vi "ETRONzipSummary.vi"() -> ()   [LabVIEW 2012]
uses:
  <vilib>/addons/database/Connection.llb/DB Tools Open Connec (Path).vi
  <vilib>/addons/database/Connection.llb/Conn Execute.vi
  <vilib>/addons/database/Recordset.llb/Rec Fetch Integer Data (R).vi
  <vilib>/addons/database/Recordset.llb/Rec Destroy - Connection.vi
  <vilib>/Utility/SMTP/NI_SMTPEmail.lvlib
  <vilib>/addons/database/NI_Database_API.lvlib
panel:
  out "concatenated string":string
  out "error out":errorcluster
  out "error out 3":errorcluster
  in  "MIME content-type (application/octet-stream)":string="application/octet-stream"
  out "error out 2":errorcluster
  out "last mod":timestamp
  in  "path":path=path "C:/temp/ETRON"
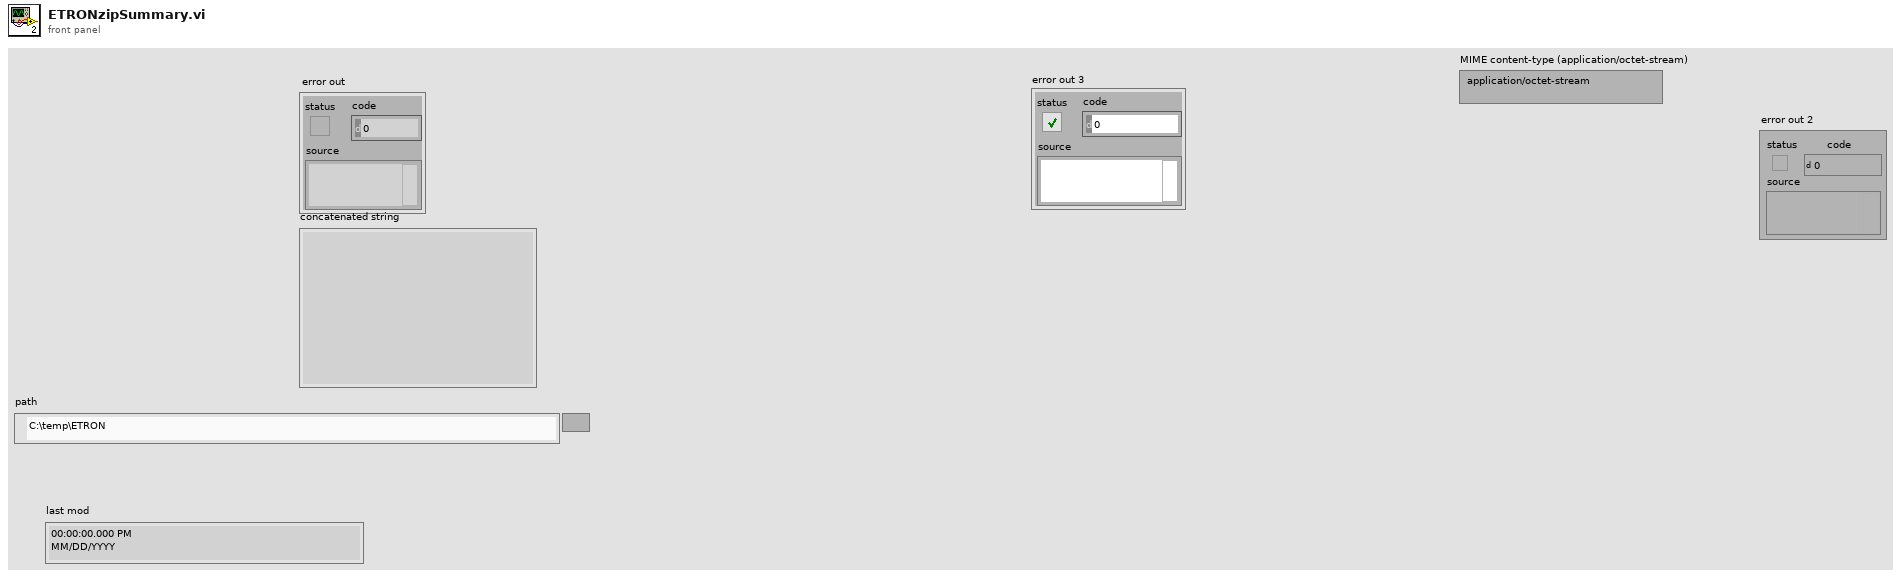
[diagram p1: front panel]
types:
  T1 = typedef "NI_Database_API.lvlib/Conn ObjectReference.ctl" = refnum<k1>
  T2 = typedef "NI_Database_API.lvlib/Rec ObjectReference.ctl" = refnum<k1>
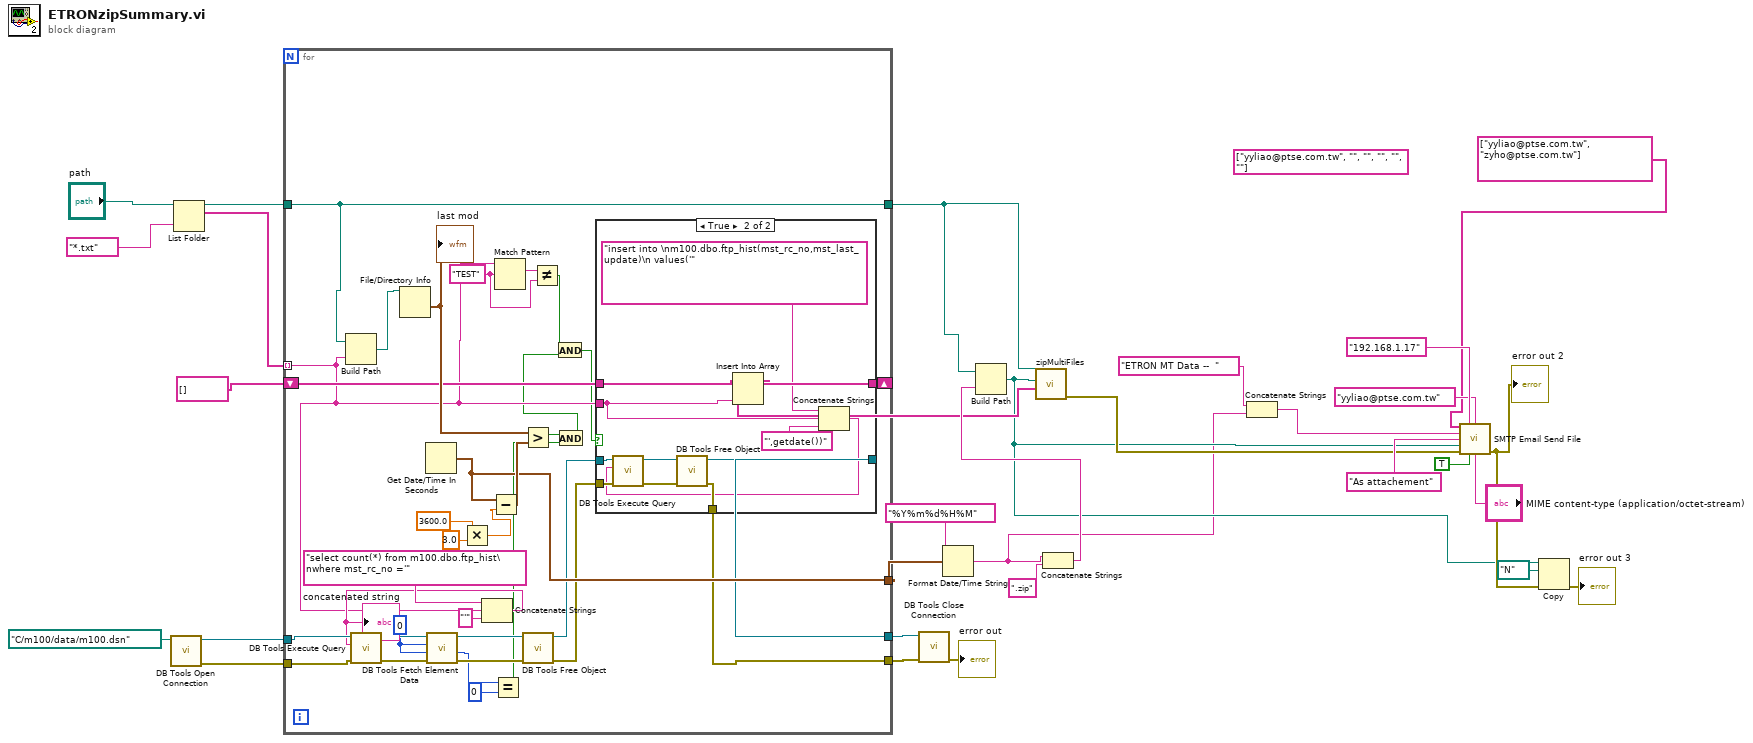
[diagram p0: block diagram]
diagram:
  (unwired) string[] ["yyliao@ptse.com.tw", "", "", "", "", ""] ("recipients")
  n1 = call-poly <vilib>:"DB Tools Open Connection.vi"("connection information"=path "C:/m100/data/m100.dsn") -> ("error out"=w6:errorcluster, "connection reference"=w7:T1)  [unwired: 7 in]
  n2 = List Folder(path="path", pattern="*.txt") -> (filenames=w28:string[])  [unwired: 2 in, 3 out]
  n3 = for {
    tunnel: "path" -> [w56]
    tunnel: w28 -> [w34] mode=indexing
    shift-right: [w58] -> w24
    shift-left: string[] [] ("array") -> [w57]
    tunnel: [w56] -> w23
    tunnel: [w55] -> w22
    tunnel: w7 -> [w52]
    tunnel: w6 -> [w51]
    tunnel: [w46] -> w5
    tunnel: [w45] -> w4
    w35 = "TEST" ("regular expression")
    w41 = 0
    n4 = Build Path(base path=w56, name or relative path=w34) -> (appended path=w59:path)
    n5 = File/Directory Info(path=w59) -> (last mod=w61:timestamp)  [unwired: 1 in, 6 out]
    "last mod" <- w61
    n6 = Get Date/Time In Seconds() -> (seconds since 1Jan1904=w55:timestamp)
    n7 = Multiply(x=3600.0, y=3.0) -> (x*y=w63:dbl)
    n8 = Concatenate Strings("select count(*) from m100.dbo.ftp_hist\nwhere mst_rc_no ='", w34, "'" ("string")) -> (w42:string)
    "concatenated string" <- w42
    n9 = call-poly <vilib>:"DB Tools Execute Query.vi"("error in (no error)"=w51, "SQL query"=w42, "connection reference"=w52) -> ("error out"=w50:errorcluster, "recordset reference"=w54:T2)  [unwired: 5 in]
    n10 = call-poly <vilib>:"DB Tools Fetch Element Data.vi"("error in (no error)"=w50, "type"=w41, "column index"=w41, "recordset reference"=w54) -> ("error out"=w49:errorcluster, "data"=w40:i32, "recordset reference out"=w53:T2)  [unwired: 3 in]
    n11 = Subtract(x=w55, y=w63) -> (x-y=w60:timestamp)
    n12 = Equal?(x=w40, y=0) -> (x = y?=w37:bool)
    n13 = Match Pattern(string=w34, regular expression=w35) -> (match substring=w36:string)  [unwired: 1 in, 3 out]
    n14 = Greater?(x=w61, y=w60) -> (0:w38:bool)
    n15 = call-poly <vilib>:"DB Tools Free Object.vi"("error in (no error)"=w49, "recordset reference"=w53) -> ("error out"=w47:errorcluster, "connection reference"=w48:T1)  [unwired: 8 in]
    n16 = Not Equal?(x=w36, y=w35) -> (x != y?=w33:bool)
    n17 = And(x=w38, y=w37) -> (x .and. y?=w31:bool)
    n18 = And(x=w33, y=w31) -> (x .and. y?=w32:bool)
    n19 = case shown="True" w32 {
      tunnel: w34 -> [_ w68]
      tunnel: [w67 w79] -> w58
      tunnel: w57 -> [w67 w78]
      tunnel: w48 -> [w66 w77]
      tunnel: w47 -> [w65 w76]
      tunnel: [w66 w72] -> w46
      tunnel: [w65 w73] -> w45
      frame False {
      }
      frame True {
        n20 = Insert Into Array(array=w78, new element=w68) -> (w79:string[])  [unwired: 1 in]
        n21 = Concatenate Strings("insert into \nm100.dbo.ftp_hist(mst_rc_no,mst_last_update)\n values('", w68, "',getdate())" ("string")) -> (w69:string)
        n22 = call-poly <vilib>:"DB Tools Execute Query.vi"("error in (no error)"=w76, "SQL query"=w69, "connection reference"=w77) -> ("error out"=w74:errorcluster, "recordset reference"=w75:T2)  [unwired: 5 in]
        n23 = call-poly <vilib>:"DB Tools Free Object.vi"("error in (no error)"=w74, "recordset reference"=w75) -> ("error out"=w73:errorcluster, "connection reference"=w72:T1)  [unwired: 8 in]
      }
    }
  }
  n24 = call <vilib>:"DB Tools Close Connection.vi"("error in (no error)"=w4, "connection reference"=w5) -> ("error out"=→"error out":errorcluster)  [unwired: 5 in]
  n25 = Format Date/Time String(time format string (%c)="%Y%m%d%H%M", seconds (now)=w22) -> (date/time string=w8:string)  [unwired: 1 in]
  n26 = Concatenate Strings(w8, ".zip" ("string")) -> (w26:string)
  n27 = Build Path(base path=w23, name or relative path=w26) -> (appended path=w12:path)
  n28 = call "zipMultiFiles.vi"("Source Files"=w24, "zip folderFile"=w12, "Source path"=w23) -> ("error out"=w13:errorcluster)  [unwired: 8 in]
  n29 = Concatenate Strings("ETRON MT Data --  " ("subject ([No Subject])"), w8) -> (w10:string)
  n30 = call <vilib>:"SMTP Email Send File.vi"("recipients"=string[] ["yyliao@ptse.com.tw", "zyho@ptse.com.tw"], "mail server"="192.168.1.17", "return address"="yyliao@ptse.com.tw", "subject ([No Subject])"=w10, "message"="As attachement", "file path"=w12, "error in (no error)"=w13, "binary? (F)"=TRUE, "MIME content-type (application/octet-stream)"="MIME content-type (application/octet-stream)") -> ("error out"=w14:errorcluster)  [unwired: 5 in, 1 out]
  "error out 2" <- w14
  n31 = Copy(8:w14, 10:path "N:/" ("target path (use dialog)"), 11:w12) -> (0:→"error out 3":errorcluster)  [unwired: 2 in, 2 out]
